vi "Programmatically Save Control Values 86 Updated 2016 09 for LV12 withXctl.vi"() -> ()   [LabVIEW 2012]
uses:
  QFingerStuff/uberkeeper-demo LV12 Folder/xcontrol-graph/ubergraphing-xcontrol.xctl
panel:
  out "ubergraphing-xcontrol":T1(xcontrol)
  in  "ColorScheme":i32
  in  "Numeric 2":dbl
  in  "STOP":bool
  in  "String":string="test"
  in  "Boolean 2":bool=TRUE
  in  "Numeric":dbl=35.0
  in  "Boolean":bool=TRUE
  in  "LOAD":bool
  in  "SAVE":bool
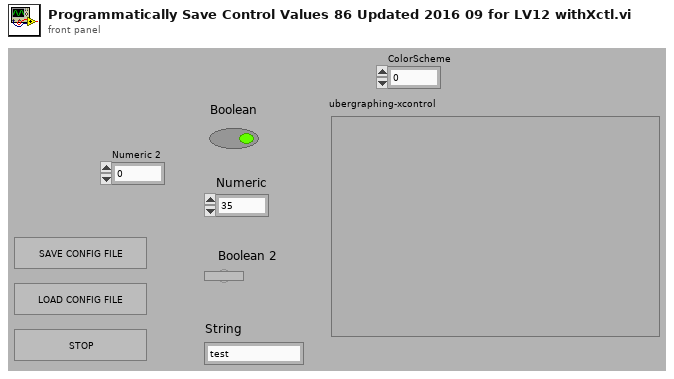
[diagram p1: front panel]
types:
  T1 = cluster{"Data Array 2D":dbl[][], "DataNames":string[]}
  T2 = cluster{"Data Array":dbl[][], "Data Names":string[]}
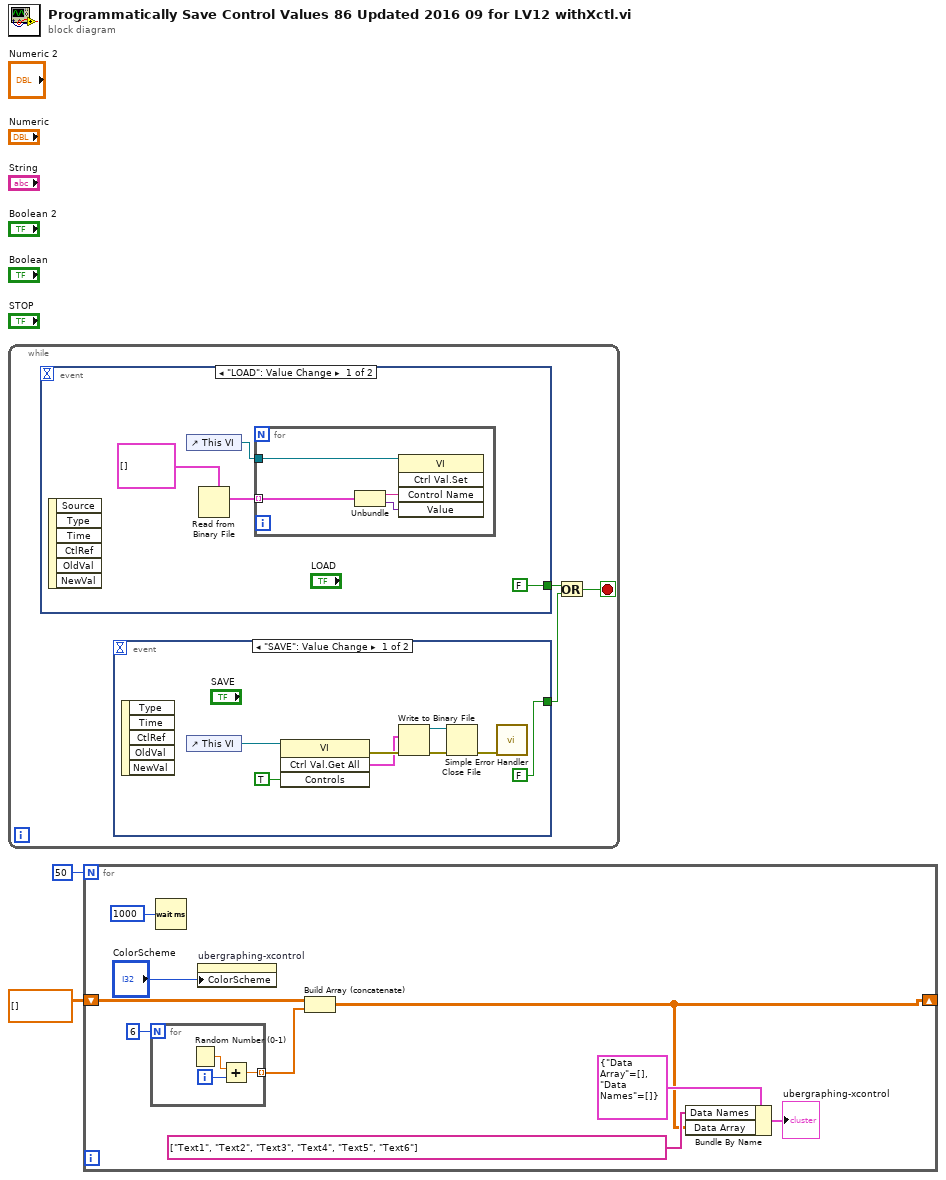
[diagram p0: block diagram]
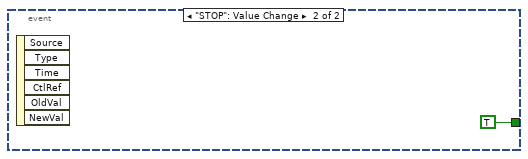
[diagram p2: hidden frame]
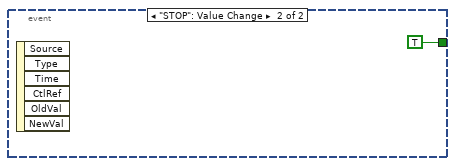
[diagram p3: hidden frame]
diagram:
  n1 = while {
    stop <- w4 stop-if-true
    n2 = event shown="[0] \"LOAD\": Value Change" {
      selector: _ -> [_ _]
      dyn-events: _ -> [_ _]
      timeout: _ -> [_ _]
      tunnel: [FALSE TRUE] -> w5
      event "LOAD": Value Change {
        n3 = event-data() -> ()  [unwired: 7 out]
        n4 = control-ref of="This VI"() -> (w9:refnum<vi>)
        n5 = Read from Binary File(5:cluster{"Name":string, "Variant Data":variant}[] [] ("Control Value:Get All")) -> (2:w6:cluster{"Name":string, "Variant Data":variant}[])  [unwired: 5 in, 3 out]
        n6 = for {
          tunnel: w9 -> [w13]
          tunnel: w6 -> [w12] mode=indexing
          n7 = Unbundle(w12) -> ("Name"=w11:string, "Variant Data"=w10:variant)
          n8 = invoke class="VI" method="Ctrl Val.Set"(reference=w13, "Control Name"=w11, "Value"=w10) -> ()  [unwired: 2 in, 5 out]
        }
      }
      event "STOP": Value Change {
        n9 = event-data() -> ()  [unwired: 7 out]
      }
    }
    n10 = event shown="[0] \"SAVE\": Value Change" {
      selector: _ -> [_ _]
      dyn-events: _ -> [_ _]
      timeout: _ -> [_ _]
      tunnel: [FALSE TRUE] -> w3
      event "SAVE": Value Change {
        n11 = event-data() -> ()  [unwired: 6 out]
        n12 = control-ref of="This VI"() -> (w21:refnum<vi>)
        n13 = invoke class="VI" method="Ctrl Val.Get All"(reference=w21, "Controls"=TRUE) -> (error out=w18:errorcluster, "Get All Control Values Variant"=w17:cluster{"Name":string, "Variant Data":variant}[])  [unwired: 2 in, 2 out]
        n14 = Write to Binary File(data=w17, error in=w18) -> (refnum out=w15:refnum<file>, error out=w16:errorcluster)  [unwired: 4 in, 1 out]
        n15 = Close File(refnum=w15, error in=w16) -> (error out=w20:errorcluster)  [unwired: 1 out]
        n16 = call <vilib>:"Simple Error Handler.vi"("error in (no error)"=w20) -> ()  [unwired: 1 in, 8 out]
      }
      event "STOP": Value Change {
        n17 = event-data() -> ()  [unwired: 7 out]
      }
    }
    n18 = Or(x=w5, y=w3) -> (x .or. y?=w4:bool)
  }
  n19 = for {
    N: 50 -> [_]
    shift-right: [w26] -> _
    shift-left: dbl[][] [] ("Data Array") -> [w29]
    n20 = for {
      N: 6 -> [_]
      tunnel: [w33] -> w28 mode=indexing
      i -> [w34]
      n21 = Random Number (0-1)() -> (number: 0 to 1=w35:dbl)
      n22 = Add(x=w35, y=w34) -> (x+y=w33:dbl)
    }
    n23 = Wait (ms)(milliseconds to wait=u32 1000) -> ()  [unwired: 1 out]
    n24 = property on="ubergraphing-xcontrol" class="ubergraphing-xcontrol (strict)"("ColorScheme"="ColorScheme") -> ()  [unwired: 2 in, 2 out]
    n25 = Build Array (concatenate)(w29, w28) -> (w26:dbl[][])
    n26 = Bundle By Name(cluster=T2 {"Data Array"=[], "Data Names"=[]} ("Data In"), "Data Names"=string[] ["Text1", "Text2", "Text3", "Text4", "Text5", "Text6"], "Data Array"=w26) -> (→"ubergraphing-xcontrol":T2)
  }
